vi "ad discrete inv.vi"(0 "adh":i32, 1 "datav":u64[](array[numeric])=array[4097 elements], 5 "chac":i32, 7 "chav":i32[](array[numeric])=array[4097 elements], 9 "rangev":u64[](array[numeric])=array[4097 elements], 11 "error in (no error)":errorcluster) -> (3 "datav out":u64[](array[numeric]), 4 "function return":i32, 15 "error out":errorcluster)   [LabVIEW 2021, in "libad4.lvlib"]
doc: "LIBAD4 function: ad_discrete_inv (int32_t adh, int32_t chac, int32_t chav[], uint64_t rangev[], uint64_t datav[]);\n\nAllows discrete values, from multiple channels, to be read from the DAQ. These value can be converted to a voltage representation via `ad_sample_to_float`.\nNote: the channel numbers must be constructed as follows `AD_CHA_TYPE_ANALOG_IN | 0x0001`, where `|` is the bitwise OR operation. The full list of prefixes are shown here: \n\nAD_CHA_TYPE_ANALOG_IN 0x01000000\nAD_CHA_TYPE_ANALOG_OUT 0x02000000\nAD_CHA_TYPE_DIGITAL_IO 0x03000000\nAD_CHA_TYPE_SYNC 0x05000000\nAD_CHA_TYPE_ROUTE 0x06000000\nAD_CHA_TYPE_CAN 0x07000000\nAD_CHA_TYPE_COUNTER 0x08000000\nAD_CHA_TYPE_ANALOG_COUNTER 0x09000000\n\nNote: 'cha constructor.vi' can be used to help calculate these values within labview."
uses:
  <userlib>/libad4/libad4.lvlib
  <userlib>/libad4/libad4.dll
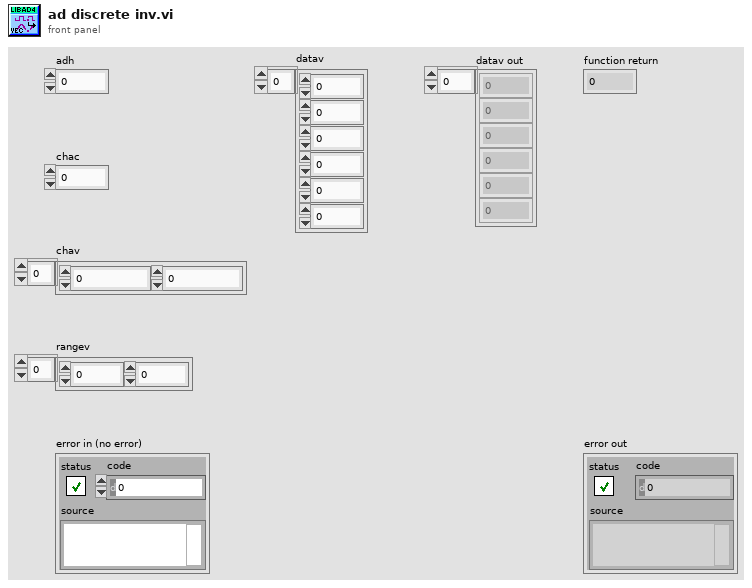
[diagram p1: front panel]
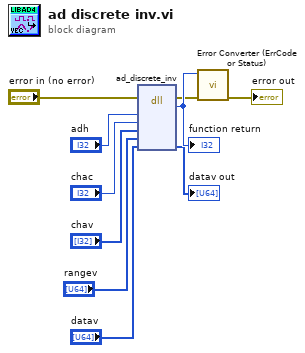
[diagram p0: block diagram]
diagram:
  n1 = dll-call lib="C:/Program Files/National Instruments/LabVIEW 2021/user.lib/libad4/libad4.*" fn="ad_discrete_inv"(error in="error in (no error)", "adh"="adh", "chac"="chac", "chav"="chav", "rangev"="rangev", "datav"="datav") -> (error out=w7:errorcluster, "return type"=w10:i32, "datav"=→"datav out":u64[])  [unwired: 6 in, 1 out]
  "function return" <- w10
  n2 = call <userlib>:"Error Converter (ErrCode or Status).vi"("error in (no error)"=w7, "error code"=w10) -> ("error out"=→"error out":errorcluster)  [unwired: 9 in]
